vi "Format Log Data.vi"(8 "error in (no error)":errorcluster, 9 "Channels":waveform(dbl)[](array[waveform]), 11 "Data Logger Module in":refnum<class "Data Logger Module.lvclass">) -> (0 "error out":errorcluster, 1 "Data":dbl[][](array[numeric]), 2 "Time":i64[](array[numeric]), 3 "Data Logger Module out":refnum<class "Data Logger Module.lvclass">)   [LabVIEW 2020, in "VolatusData.lvlib" / "Data Logger Module.lvclass"]
uses:
  Data Logger Module.lvclass
  Data Logger Module.lvclass/Data Logger Module.ctl
  lv-vecto/Vecto/Vecto.lvlib
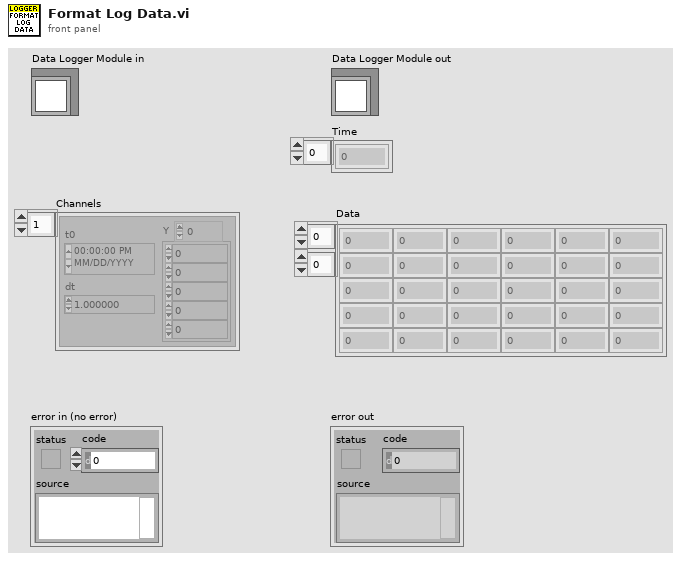
[diagram p1: front panel]
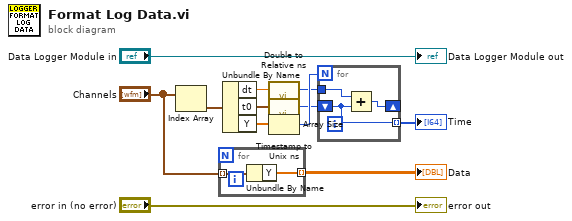
[diagram p0: block diagram]
diagram:
  n1 = Index Array(array="Channels") -> (element=w10:waveform(dbl))  [unwired: 1 in]
  n2 = for {
    tunnel: "Channels" -> [w14] mode=indexing
    tunnel: [w13] -> w6 mode=indexing
    n3 = Unbundle By Name(w14) -> ("Y"=w13:dbl[])
  }
  "Data" <- w6
  n4 = Unbundle By Name(w10) -> ("dt"=w5:dbl, "t0"=w4:timestamp, "Y"=w9:dbl[])
  n5 = call "Double to Relative ns.vi"("Double"=w5) -> ("Relative ns"=w2:i64)  [unwired: 2 in]
  n6 = call "Timestamp to Unix ns.vi"("Time Stamp"=w4) -> ("unix ns"=w3:i64)  [unwired: 2 in]
  n7 = Array Size(array=w9) -> (size(s)=w8:i32)
  n8 = for {
    N: w8 -> [_]
    shift-right: [w15] -> _
    shift-left: w3 -> [w17]
    tunnel: w2 -> [w16]
    tunnel: [w17] -> w1 mode=indexing
    n9 = Add(x=w16, y=w17) -> (x+y=w15:i64)
  }
  "Time" <- w1
  "error out" <- "error in (no error)"
  "Data Logger Module out" <- "Data Logger Module in"
